vi "json_parse_value.vi"(7 "elements in":T1[](array[typedef]), 8 "error in (no error)":errorcluster, 9 "offset (0)":i32, 10 "path":string, 11 "data":string) -> (0 "error out":errorcluster, 1 "offset past match":i32, 2 "elements out":T1[](array[typedef]))   [LabVIEW 2017]
uses:
  json_element.ctl
  json_element_type.ctl
  <vilib>/regexp/Match Regular Expression.xnode
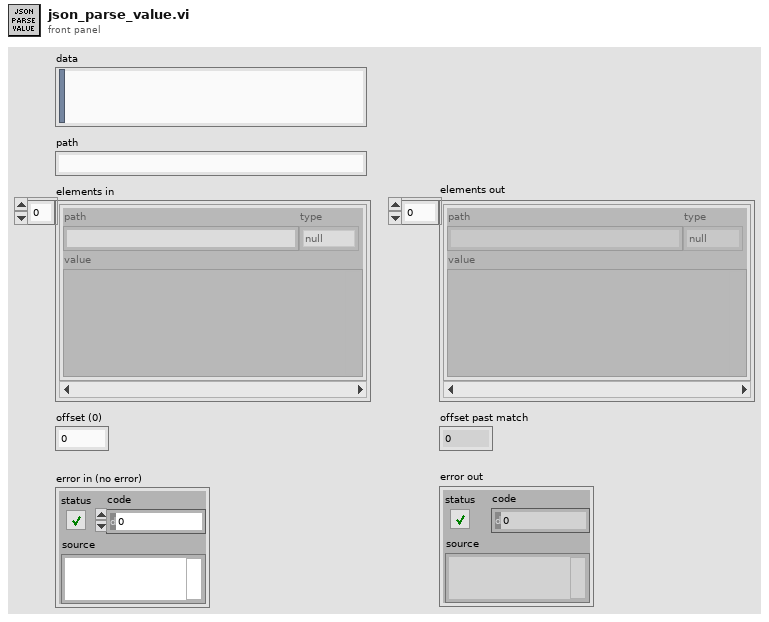
[diagram p1: front panel]
types:
  T1 = typedef "json_element.ctl" = cluster{"path":string, "type":T2, "value":variant}
  T2 = typedef "json_element_type.ctl" = enum8{"null", "bool", "int", "uint", "float", "string", "array", "object"}
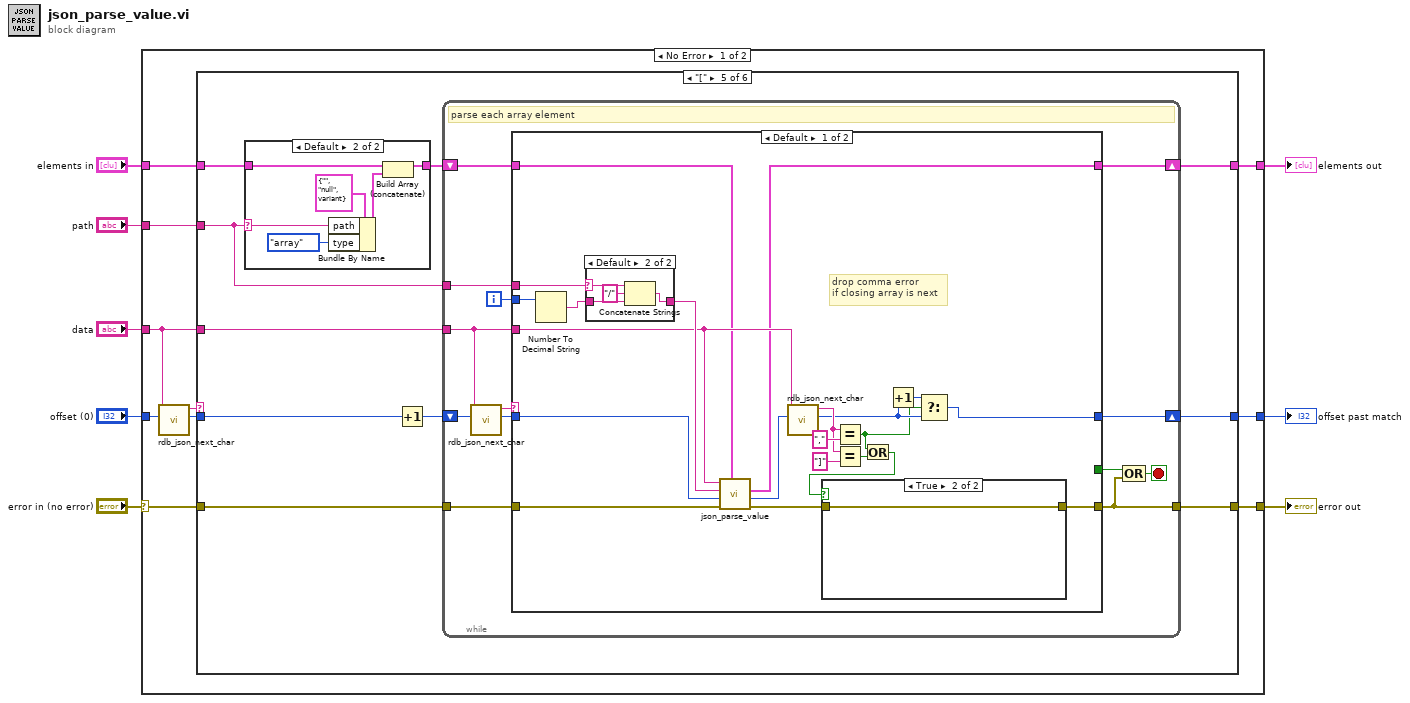
[diagram p0: block diagram]
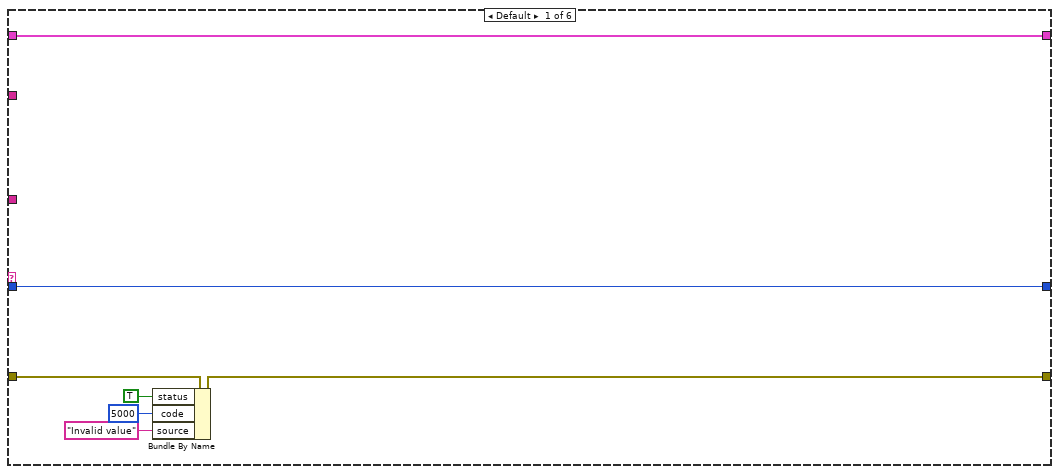
[diagram p2: hidden frame]
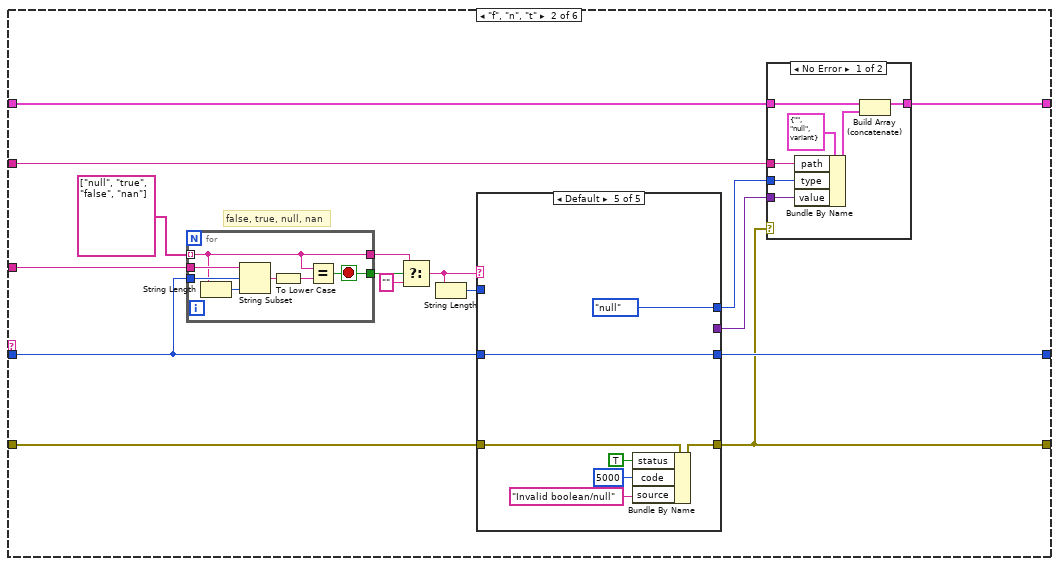
[diagram p3: hidden frame]
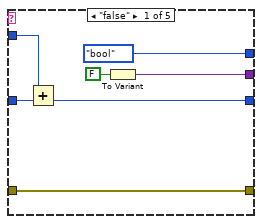
[diagram p4: hidden frame]
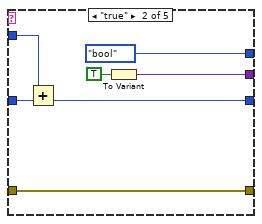
[diagram p5: hidden frame]
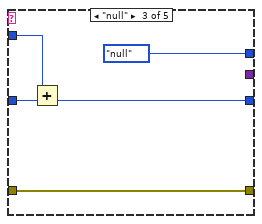
[diagram p6: hidden frame]
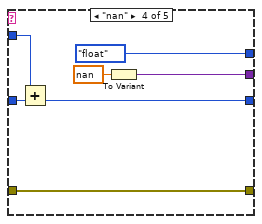
[diagram p7: hidden frame]
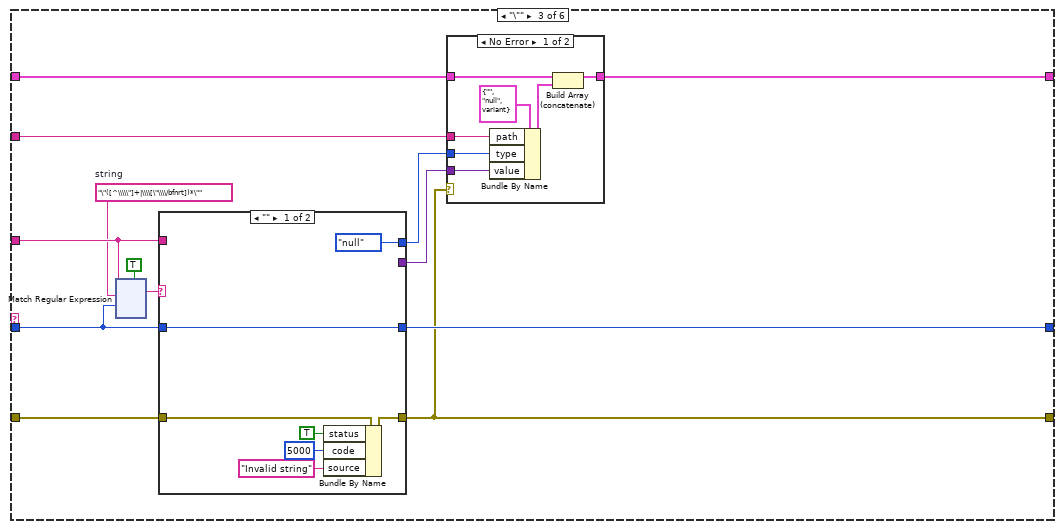
[diagram p9: hidden frame]
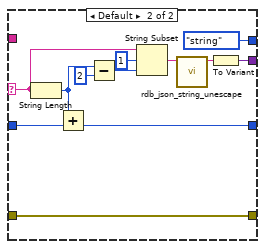
[diagram p11: hidden frame]
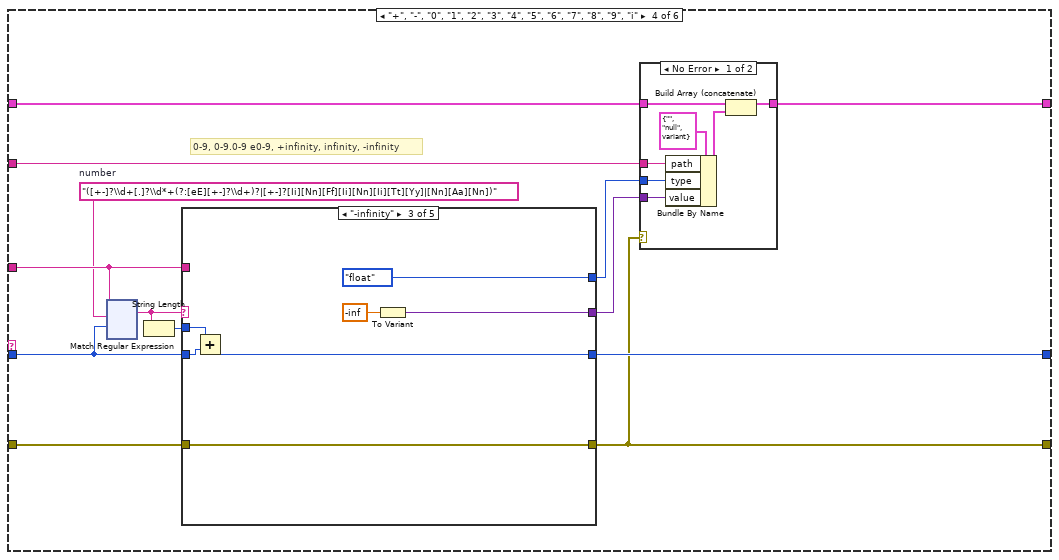
[diagram p12: hidden frame]
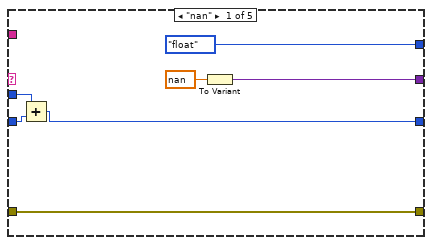
[diagram p14: hidden frame]
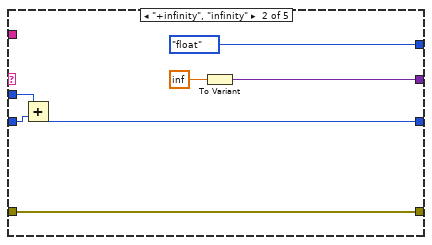
[diagram p15: hidden frame]
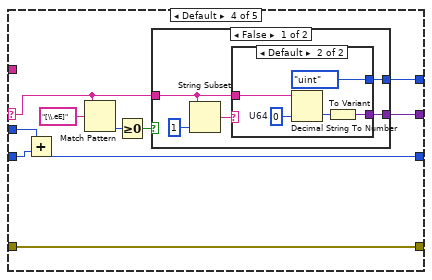
[diagram p16: hidden frame]
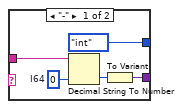
[diagram p17: hidden frame]
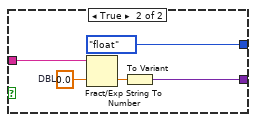
[diagram p18: hidden frame]
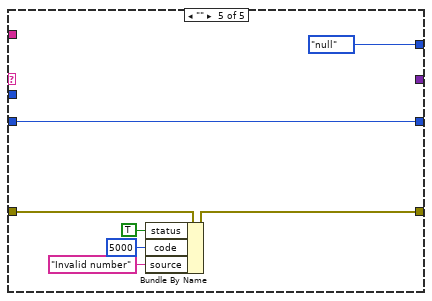
[diagram p19: hidden frame]
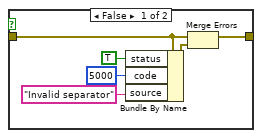
[diagram p20: hidden frame]
diagram:
  n1 = case shown="No Error" "error in (no error)" {
    selector: "error in (no error)" -> [w16 w591]
    tunnel: [w18 w589] -> w8
    tunnel: "path" -> [w17 _]
    tunnel: "data" -> [w12 _]
    tunnel: [w15 w591] -> w4
    tunnel: "offset (0)" -> [w13 w590]
    tunnel: [w14 w590] -> w2
    tunnel: "elements in" -> [w10 w589]
    frame No Error {
      n2 = call "rdb_json_next_char.vi"("offset (0)"=w13, "json"=w12) -> ("offset before char"=w11:i32, "non-whitespace char"=w9:string)  [unwired: 8 in]
      n3 = case shown="\"[\"" w9 {
        tunnel: [w22 w41 w91 w245 w446 w514] -> w18
        tunnel: w17 -> [_ w40 w94 w248 w440 w508]
        tunnel: w16 -> [w25 w37 w102 w256 w445 w513]
        tunnel: [w24 w35 w92 w246 w444 w512] -> w15
        tunnel: [w23 w36 w99 w254 w443 w511] -> w14
        tunnel: w12 -> [_ w39 w101 w253 w441 w509]
        tunnel: w11 -> [w23 w38 w100 w255 w442 w510]
        tunnel: w10 -> [w22 w34 w95 w249 w437 w507]
        frame Default {
          n4 = Bundle By Name(cluster=w25, "status"=TRUE, "code"=5000, "source"="Invalid value") -> (w24:errorcluster)
        }
        frame "f", "n", "t" {
          # "false, true, null, nan"
          n5 = for {
            tunnel: w39 -> [w81]
            tunnel: w38 -> [w80]
            tunnel: string[] ["null", "true", "false", "nan"] -> [w75] mode=indexing
            tunnel: [w76] -> w31
            tunnel: [w75] -> w30
            stop <- w76 stop-if-true
            n6 = String Length(string=w75) -> (length=w77:i32)
            n7 = String Subset(string=w81, offset (0)=w80, length (rest)=w77) -> (substring=w79:string)
            n8 = To Lower Case(string=w79) -> (all lower case string=w78:string)
            n9 = Equal?(x=w75, y=w78) -> (x = y?=w76:bool)
          }
          n10 = Select(t=w30, s=w31, f="") -> (s? t:f=w28:string)
          n11 = String Length(string=w28) -> (length=w27:i32)
          n12 = case shown="Default" w28 {
            tunnel: [w43 w50 w57 w63 w74] -> w35
            tunnel: w37 -> [w43 w50 w57 w63 w73]
            tunnel: [w47 w54 _ w67 _] -> w33
            tunnel: [w45 w52 w59 w65 w69] -> w36
            tunnel: w38 -> [w46 w53 w60 w66 w69]
            tunnel: w27 -> [w44 w51 w58 w64 _]
            tunnel: [json_element_type."bool" ("type") json_element_type."bool" ("type") json_element_type."null" ("type") json_element_type."float" ("type") json_element_type."null" ("type")] -> w26
            frame "false" {
              n13 = Add(x=w44, y=w46) -> (x+y=w45:i32)
              n14 = To Variant(anything=FALSE) -> (Variant=w47:variant)
            }
            frame "true" {
              n15 = Add(x=w51, y=w53) -> (x+y=w52:i32)
              n16 = To Variant(anything=TRUE) -> (Variant=w54:variant)
            }
            frame "null" {
              n17 = Add(x=w58, y=w60) -> (x+y=w59:i32)
            }
            frame "nan" {
              n18 = Add(x=w64, y=w66) -> (x+y=w65:i32)
              n19 = To Variant(anything=nan) -> (Variant=w67:variant)
            }
            frame Default {
              n20 = Bundle By Name(cluster=w73, "status"=TRUE, "code"=5000, "source"="Invalid boolean/null") -> (w74:errorcluster)
            }
          }
          n21 = case shown="No Error" w35 {
            tunnel: w33 -> [w87 _]
            tunnel: w40 -> [w88 _]
            tunnel: [w85 w89] -> w41
            tunnel: w34 -> [w84 w89]
            tunnel: w26 -> [w82 _]
            frame No Error {
              n22 = Bundle By Name(cluster=T1 {"path"="", "type"=enum."null", "value"=variant} ("element"), "path"=w88, "type"=w82, "value"=w87) -> (w86:T1)
              n23 = Build Array (concatenate)(w84, w86) -> (w85:T1[])
            }
            frame Error {
            }
          }
        }
        frame "\"" {
          w98 = "\"([^\\\\\"]+|\\\\[\"\\\\/bfnrt])*\""  # string
          n24 = xnode ("Match Regular Expression")("input string"=w101, "regular expression"=w98, "offset (0)"=w100, "multiline? (F)"=TRUE) -> ("whole match"=w96:string)  [unwired: 2 in, 4 out]
          n25 = case shown="\"\"" w96 {
            selector: w96 -> [_ w122]
            tunnel: w101 -> [_ _]
            tunnel: [_ w127] -> w93
            tunnel: [w116 w123] -> w92
            tunnel: w102 -> [w117 w123]
            tunnel: w100 -> [w112 w121]
            tunnel: [w112 w120] -> w99
            tunnel: [json_element_type."null" ("type") json_element_type."string" ("type")] -> w90
            frame "" {
              n26 = Bundle By Name(cluster=w117, "status"=TRUE, "code"=5000, "source"="Invalid string") -> (w116:errorcluster)
            }
            frame Default {
              n27 = String Length(string=w122) -> (length=w119:i32)
              n28 = Add(x=w119, y=w121) -> (x+y=w120:i32)
              n29 = Subtract(x=w119, y=2) -> (x-y=w124:i32)
              n30 = String Subset(string=w122, offset (0)=1, length (rest)=w124) -> (substring=w129:string)
              n31 = call "rdb_json_string_unescape.vi"("escaped string"=w129) -> ("string out"=w128:string)  [unwired: 9 in, 1 out]
              n32 = To Variant(anything=w128) -> (Variant=w127:variant)
            }
          }
          n33 = case shown="No Error" w92 {
            tunnel: w93 -> [w108 _]
            tunnel: w94 -> [w109 _]
            tunnel: [w106 w110] -> w91
            tunnel: w95 -> [w105 w110]
            tunnel: w90 -> [w103 _]
            frame No Error {
              n34 = Bundle By Name(cluster=T1 {"path"="", "type"=enum."null", "value"=variant} ("element"), "path"=w109, "type"=w103, "value"=w108) -> (w107:T1)
              n35 = Build Array (concatenate)(w105, w107) -> (w106:T1[])
            }
            frame Error {
            }
          }
        }
        frame "+", "-", "0", "1", "2", "3", "4", "5", "6", "7", "8", "9", "i" {
          w252 = "([+-]?\\d+[.]?\\d*+(?:[eE][+-]?\\d+)?|[+-]?[Ii][Nn][Ff][Ii][Nn][Ii][Tt][Yy]|[Nn][Aa][Nn])"  # number
          # "0-9, 0-9.0-9 e0-9, +infinity, infinity, -infinity"
          n36 = xnode "Match Regular Expression"("input string"=w253, "regular expression"=w252, "offset (0)"=w255) -> ("whole match"=w251:string)  [unwired: 3 in, 4 out]
          n37 = String Length(string=w251) -> (length=w250:i32)
          n38 = case shown="\"-infinity\"" w251 {
            selector: w251 -> [_ _ _ w290 _]
            tunnel: [w270 w277 w284 w295 _] -> w247
            tunnel: [w269 w276 w283 w291 w318] -> w246
            tunnel: w256 -> [w269 w276 w283 w291 w319]
            tunnel: w253 -> [_ _ _ _ _]
            tunnel: w255 -> [w268 w275 w282 w289 w317]
            tunnel: [w267 w274 w281 w288 w317] -> w254
            tunnel: w250 -> [w266 w273 w280 w287 _]
            tunnel: [json_element_type."float" ("type") json_element_type."float" ("type") json_element_type."float" ("type") w286 json_element_type."null" ("type")] -> w244
            frame "nan" {
              n39 = Add(x=w266, y=w268) -> (x+y=w267:i32)
              n40 = To Variant(anything=nan) -> (Variant=w270:variant)
            }
            frame "+infinity", "infinity" {
              n41 = Add(x=w273, y=w275) -> (x+y=w274:i32)
              n42 = To Variant(anything=inf) -> (Variant=w277:variant)
            }
            frame "-infinity" {
              n43 = Add(x=w280, y=w282) -> (x+y=w281:i32)
              n44 = To Variant(anything=-inf) -> (Variant=w284:variant)
            }
            frame Default {
              n45 = Add(x=w287, y=w289) -> (x+y=w288:i32)
              n46 = Match Pattern(string=w290, regular expression="[\\.eE]") -> (offset past match=w293:i32)  [unwired: 1 in, 3 out]
              n47 = Greater Or Equal To 0?(x=w293) -> (x >= 0?=w292:bool)
              n48 = case shown="False" w292 {
                tunnel: w290 -> [w299 w315]
                tunnel: [w298 w312] -> w295
                tunnel: [w296 json_element_type."float" ("type")] -> w286
                frame False {
                  n49 = String Subset(string=w299, length (rest)=1 ("length (rest)")) -> (substring=w297:string)  [unwired: 1 in]
                  n50 = case shown="Default" w297 {
                    tunnel: w299 -> [w305 w310]
                    tunnel: [w302 w307] -> w298
                    tunnel: [json_element_type."int" ("type") json_element_type."uint" ("type")] -> w296
                    frame "-" {
                      w304 = i64 0  # I64
                      n51 = Decimal String To Number(string=w305, default (0L)=w304) -> (number=w303:i64)  [unwired: 1 in, 1 out]
                      n52 = To Variant(anything=w303) -> (Variant=w302:variant)
                    }
                    frame Default {
                      w309 = u64 0  # U64
                      n53 = Decimal String To Number(string=w310, default (0L)=w309) -> (number=w308:u64)  [unwired: 1 in, 1 out]
                      n54 = To Variant(anything=w308) -> (Variant=w307:variant)
                    }
                  }
                }
                frame True {
                  w314 = 0.0  # DBL
                  n55 = Fract/Exp String To Number(string=w315, default (0 dbl)=w314) -> (number=w313:dbl)  [unwired: 2 in, 1 out]
                  n56 = To Variant(anything=w313) -> (Variant=w312:variant)
                }
              }
            }
            frame "" {
              n57 = Bundle By Name(cluster=w319, "status"=TRUE, "code"=5000, "source"="Invalid number") -> (w318:errorcluster)
            }
          }
          n58 = case shown="No Error" w246 {
            tunnel: w247 -> [w262 _]
            tunnel: w248 -> [w263 _]
            tunnel: [w260 w264] -> w245
            tunnel: w249 -> [w259 w264]
            tunnel: w244 -> [w257 _]
            frame No Error {
              n59 = Bundle By Name(cluster=T1 {"path"="", "type"=enum."null", "value"=variant} ("element"), "path"=w263, "type"=w257, "value"=w262) -> (w261:T1)
              n60 = Build Array (concatenate)(w259, w261) -> (w260:T1[])
            }
            frame Error {
            }
          }
        }
        frame "[" {
          n61 = case shown="Default" w440 {
            selector: w440 -> [_ w502]
            tunnel: [w498 w503] -> w439
            tunnel: w437 -> [w498 w501]
            frame "" {
            }
            frame Default {
              n62 = Bundle By Name(cluster=T1 {"path"="", "type"=enum."null", "value"=variant} ("element"), "path"=w502, "type"=json_element_type."array") -> (w504:T1)
              n63 = Build Array (concatenate)(w501, w504) -> (w503:T1[])
            }
          }
          n64 = Increment(x=w442) -> (x+1=w438:i32)
          n65 = while {
            shift-right: [w459] -> w446
            shift-left: w439 -> [w458]
            tunnel: w445 -> [w457]
            tunnel: [w453] -> w444
            tunnel: w440 -> [w456]
            tunnel: w441 -> [w449]
            shift-right: [w451] -> w443
            shift-left: w438 -> [w450]
            i -> [w452]
            stop <- w454 stop-if-true
            # "parse each array element"
            n66 = call "rdb_json_next_char.vi"("offset (0)"=w450, "json"=w449) -> ("offset before char"=w448:i32, "non-whitespace char"=w447:string)  [unwired: 8 in]
            n67 = case shown="Default" w447 {
              tunnel: [_ TRUE] -> w455
              tunnel: [w471 w496] -> w459
              tunnel: w458 -> [w472 w496]
              tunnel: w449 -> [w473 _]
              tunnel: w457 -> [w479 w495]
              tunnel: [w467 w495] -> w453
              tunnel: w456 -> [w480 _]
              tunnel: w452 -> [w477 _]
              tunnel: w448 -> [w474 w494]
              tunnel: [w463 w493] -> w451
              frame Default {
                # "drop comma error\nif closing array is next"
                n68 = Number To Decimal String(number=w477) -> (decimal integer string=w476:string)  [unwired: 1 in]
                n69 = case shown="Default" w480 {
                  selector: w480 -> [_ w492]
                  tunnel: w476 -> [w488 w491]
                  tunnel: [w488 w490] -> w478
                  frame "" {
                  }
                  frame Default {
                    n70 = Concatenate Strings(w492, "/" ("format string"), w491) -> (w490:string)
                  }
                }
                n71 = call "json_parse_value.vi"("elements in"=w472, "error in (no error)"=w479, "offset (0)"=w474, "path"=w478, "data"=w473) -> ("error out"=w466:errorcluster, "offset past match"=w468:i32, "elements out"=w471:T1[])  [unwired: 4 in]
                n72 = call "rdb_json_next_char.vi"("offset (0)"=w468, "json"=w473) -> ("offset before char"=w462:i32, "non-whitespace char"=w469:string)  [unwired: 8 in]
                n73 = Equal?(x=w469, y=",") -> (x = y?=w460:bool)
                n74 = Equal?(x=w469, y="]") -> (x = y?=w464:bool)
                n75 = Or(x=w460, y=w464) -> (x .or. y?=w465:bool)
                n76 = case shown="True" w465 {
                  tunnel: [w486 w487] -> w467
                  tunnel: w466 -> [w485 w487]
                  frame False {
                    n77 = Bundle By Name(cluster=w485, "status"=TRUE, "code"=5000, "source"="Invalid separator") -> (w484:errorcluster)
                    n78 = Merge Errors(w485, w484) -> (w486:errorcluster)
                  }
                  frame True {
                  }
                }
                n79 = Increment(x=w462) -> (x+1=w461:i32)
                n80 = Select(t=w461, s=w460, f=w462) -> (s? t:f=w463:i32)
              }
              frame "]" {
                n81 = Increment(x=w494) -> (x+1=w493:i32)
              }
            }
            n82 = Compound Arithmetic op=OR(w455, w453) -> (w454:bool)
          }
        }
        frame "{" {
          n83 = case shown="Default" w508 {
            selector: w508 -> [_ w519]
            tunnel: [w515 w520] -> w506
            tunnel: w507 -> [w515 w518]
            frame "" {
            }
            frame Default {
              n84 = Bundle By Name(cluster=T1 {"path"="", "type"=enum."null", "value"=variant} ("element"), "path"=w519, "type"=json_element_type."object") -> (w521:T1)
              n85 = Build Array (concatenate)(w518, w521) -> (w520:T1[])
            }
          }
          n86 = Increment(x=w510) -> (x+1=w505:i32)
          n87 = while {
            shift-right: [w533] -> w514
            shift-left: w506 -> [w532]
            tunnel: w513 -> [w531]
            tunnel: [w527] -> w512
            tunnel: w508 -> [w530]
            tunnel: w509 -> [w525]
            shift-right: [w526] -> w511
            shift-left: w505 -> [w524]
            stop <- w528 stop-if-true
            # "parse each \"key\":value pair"
            n88 = call "rdb_json_next_char.vi"("offset (0)"=w524, "json"=w525) -> ("offset before char"=w523:i32, "non-whitespace char"=w522:string)  [unwired: 8 in]
            n89 = case shown="Default" w522 {
              tunnel: [_ TRUE] -> w529
              tunnel: [w543 w587] -> w533
              tunnel: w532 -> [w542 w587]
              tunnel: w525 -> [w538 _]
              tunnel: w531 -> [w540 w586]
              tunnel: [w544 w586] -> w527
              tunnel: w530 -> [w541 _]
              tunnel: w523 -> [w539 w585]
              tunnel: [w537 w584] -> w526
              frame Default {
                n90 = call "rdb_json_decode_key.vi"("offset (0)"=w539, "data"=w538) -> ("error out"=w535:errorcluster, "offset past match"=w536:i32, "key"=w534:string)  [unwired: 7 in]
                n91 = case shown="No Error" w535 {
                  tunnel: [w550 w582] -> w544
                  tunnel: [w557 w578] -> w543
                  tunnel: w542 -> [w558 w578]
                  tunnel: w541 -> [w564 _]
                  tunnel: w534 -> [w563 _]
                  tunnel: w538 -> [w559 _]
                  tunnel: w540 -> [w562 w583]
                  tunnel: w536 -> [w560 w577]
                  tunnel: [w548 w577] -> w537
                  frame No Error {
                    # "drop comma error\nif closing object is next"
                    n92 = case shown="Default" w564 {
                      selector: w564 -> [_ w576]
                      tunnel: w563 -> [w572 w575]
                      tunnel: [w572 w574] -> w561
                      frame "" {
                      }
                      frame Default {
                        n93 = Concatenate Strings(w576, "/" ("format string"), w575) -> (w574:string)
                      }
                    }
                    n94 = call "json_parse_value.vi"("elements in"=w558, "error in (no error)"=w562, "offset (0)"=w560, "path"=w561, "data"=w559) -> ("error out"=w551:errorcluster, "offset past match"=w556:i32, "elements out"=w557:T1[])  [unwired: 4 in]
                    n95 = call "rdb_json_next_char.vi"("offset (0)"=w556, "json"=w559) -> ("offset before char"=w546:i32, "non-whitespace char"=w549:string)  [unwired: 8 in]
                    n96 = Equal?(x=w549, y=",") -> (x = y?=w547:bool)
                    n97 = Equal?(x=w549, y="}") -> (x = y?=w553:bool)
                    n98 = Increment(x=w546) -> (x+1=w545:i32)
                    n99 = Or(x=w547, y=w553) -> (x .or. y?=w552:bool)
                    n100 = case shown="False" w552 {
                      tunnel: [w570 w571] -> w550
                      tunnel: w551 -> [w569 w571]
                      frame False {
                        n101 = Bundle By Name(cluster=w569, "status"=TRUE, "code"=5000, "source"="Invalid separator") -> (w568:errorcluster)
                        n102 = Merge Errors(w569, w568) -> (w570:errorcluster)
                      }
                      frame True {
                      }
                    }
                    n103 = Select(t=w545, s=w547, f=w546) -> (s? t:f=w548:i32)
                  }
                  frame Error {
                    n104 = Bundle By Name(cluster=w583, "status"=TRUE, "code"=5000, "source"="Invalid key") -> (w582:errorcluster)
                  }
                }
              }
              frame "}" {
                n105 = Increment(x=w585) -> (x+1=w584:i32)
              }
            }
            n106 = Compound Arithmetic op=OR(w529, w527) -> (w528:bool)
          }
        }
      }
    }
    frame Error {
    }
  }
  "elements out" <- w8
  "error out" <- w4
  "offset past match" <- w2
